vi "ResetDAQmxTasks.vi"(11 "Array":tag[](array[tag])) -> ()   [LabVIEW 2014]
doc: "Resets DAQmx Tasks."
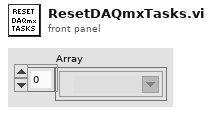
[diagram p1: front panel]
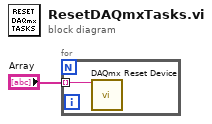
[diagram p0: block diagram]
diagram:
  n1 = for {
    tunnel: "Array" -> [w2] mode=indexing
    n2 = call <vilib>:"DAQmx Reset Device.vi"("device in"=w2) -> ()  [unwired: 14 in, 1 out]
  }
